vi "upload File to FTP.vi"(8 "error in (no error)":errorcluster, 9 "ftp path":string, 10 "Path":path, 11 "FTPProtocol in":refnum<class "FTPProtocol.lvclass">) -> (0 "error out":errorcluster, 3 "FTPProtocol out":refnum<class "FTPProtocol.lvclass">)   [LabVIEW 2020, in "FileSync -- FTP.lvlib" / "FTPProtocol.lvclass"]
uses:
  FTPProtocol.lvclass
  FTPProtocol.lvclass/FTPProtocol.ctl
  Read FTP.vi
  _support/FTP Toolkit/FTP Class/FTP.lvclass
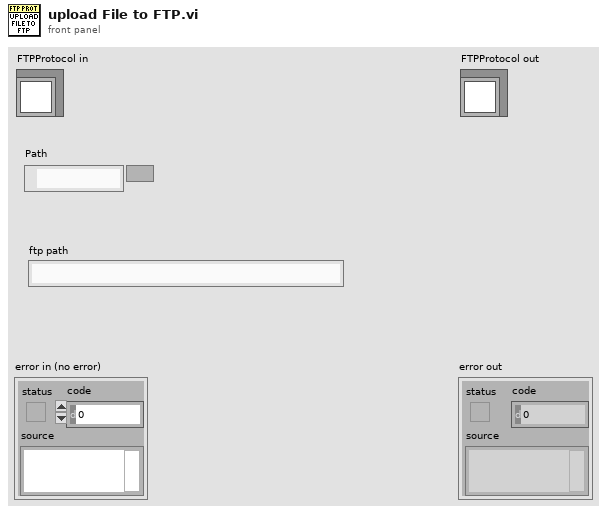
[diagram p1: front panel]
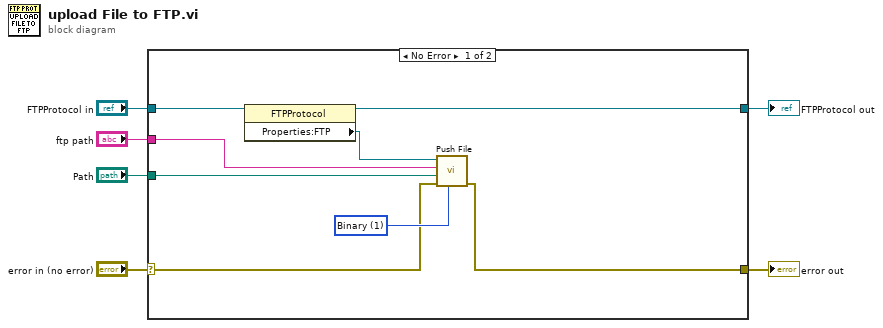
[diagram p0: block diagram]
diagram:
  n1 = case shown="No Error" "error in (no error)" {
    selector: "error in (no error)" -> [w8 w16]
    tunnel: [w7 w16] -> w5
    tunnel: [w10 w15] -> w3
    tunnel: "FTPProtocol in" -> [w14 w15]
    tunnel: "Path" -> [w12 _]
    tunnel: "ftp path" -> [w11 _]
    frame No Error {
      w13 = u16 1 items=["ASCII", "Binary"] ("Type (Binary)")
      n2 = property class="FTPProtocol"(reference=w14) -> (reference out=w10:refnum<class "FTPProtocol.lvclass">, "Properties:FTP"=w9:refnum<class "FTP.lvclass">)  [unwired: 1 in, 1 out]
      n3 = call "Push File.vi"("Type (Binary)"=w13, "error in (no error)"=w8, "Local FilePath"=w12, "Remote FileName"=w11, "FTP in"=w9) -> ("error out"=w7:errorcluster)  [unwired: 5 in, 1 out]
    }
    frame Error {
    }
  }
  "error out" <- w5
  "FTPProtocol out" <- w3
